vi "Untitled 4.vi"() -> ()   [LabVIEW 2020, in "SQLite.lvclass"]
uses:
  SQLite.lvclass
  ResultsDB/Order.ctl
  SQLite.lvclass/SQLite.ctl
panel:
  out "error out":errorcluster
  in  "Checkbox":bool
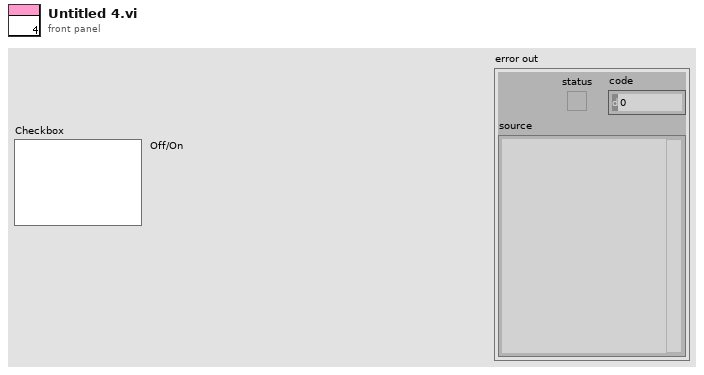
[diagram p1: front panel]
types:
  T1 = typedef "SQLite.lvclass/Order.ctl" = cluster{"OrderNum":string, "ProductNum":string, "CustomerNum":string, "EmployeeNum":string, "WorkOrder":string}
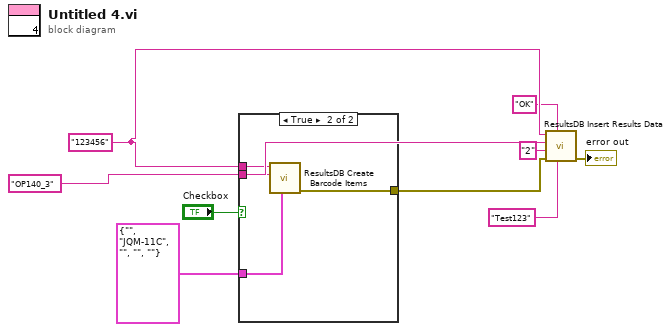
[diagram p0: block diagram]
diagram:
  w7 = "OP140_3" ("StationName")
  w8 = "123456" ("MainBarcode")
  n1 = case shown="True" "Checkbox" {
    tunnel: T1 {"OrderNum"="", "ProductNum"="JQM-11C", "CustomerNum"="", "EmployeeNum"="", "WorkOrder"=""} ("Order") -> [_ w13]
    tunnel: w8 -> [_ w12]
    tunnel: w7 -> [_ w11]
    tunnel: [_ w10] -> w3
    frame False {
    }
    frame True {
      n2 = call "ResultsDB Create Barcode Items.vi"("Order"=w13, "StationName"=w11, "MainBarcode"=w12) -> ("error out"=w10:errorcluster)  [unwired: 6 in, 2 out]
    }
  }
  n3 = call "ResultsDB Insert Results Data.vi"("Results NameList"="Test123", "Total_OK/NG"="OK", "error in (no error)"=w3, "Results List"="2", "StationName"=w7, "MainBarcode"=w8) -> ("error out"=→"error out":errorcluster)  [unwired: 4 in, 1 out]
